vi "GA_Encode.vi"(6 "Parameters":T1={"Population size"=100, "Generations no."=500, "Significant digits"=4, "Crossover probabality"=0.85, "Mutation mode"=enum."one-point, fixed rate", "Use Gray code?"=FALSE, "Mutation rate"=0.05, "Min mutation rate"=0.0005, "Max mutation rate"=0.25, "Reproduction plan"=enum."Steady-state-replace-worst", "Elitism"=FALSE, "Fmax"=1} {"Max mutation rate" min=0.0 max=1.0; "Min mutation rate" min=0.0 max=1.0; "Mutation rate" min=0.0 max=1.0; "Crossover probabality" min=0.0 max=1.0; "Significant digits" min=1; "Generations no." min=1; "Population size" min=1}, 11 "Phenotype":i32[](array[numeric])) -> (3 "Genotype":i8[](array[numeric]))   [LabVIEW 2016, in "Optimal Frequency Bands Search.lvlib" / "GeneticAlgorithm.lvlib"]
doc: "Преобразовать фенотип в генотип. Возможно кодирование генома с помощью двоичного кода, либо кода Грея"
uses:
  GeneticAlgorithm.lvlib
  GA_tParameters.ctl
panel:
  # "This VI is a part of BCI Design library, http://www.ru-bci.org \nCopyright © 2020, Sotnikov Peter, All rights reserved. License: CC BY-NC 4.0"
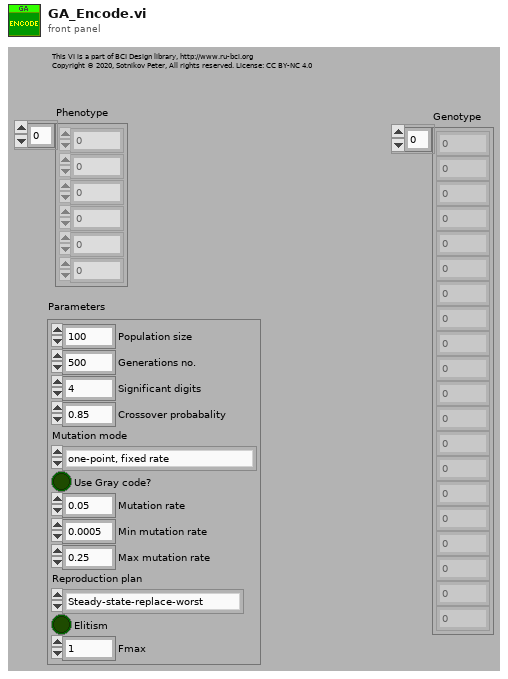
[diagram p1: front panel]
types:
  T1 = typedef "Optimal Frequency Bands Search.lvlib/GeneticAlgorithm.lvlib/GA_tParameters.ctl" = cluster{"Population size":i32, "Generations no.":i32, "Significant digits":i32, "Crossover probabality":dbl, "Mutation mode":enum16{"one-point, fixed rate", "one-point, fitness-adjustable rate", "one-point, distance-adjustable rate"}, "Use Gray code?":bool, "Mutation rate":dbl, "Min mutation rate":dbl, "Max mutation rate":dbl, "Reproduction plan":enum16{"Full generational replacement", "Steady-state-replace-random", "Steady-state-replace-worst"}, "Elitism":bool, "Fmax":i32}
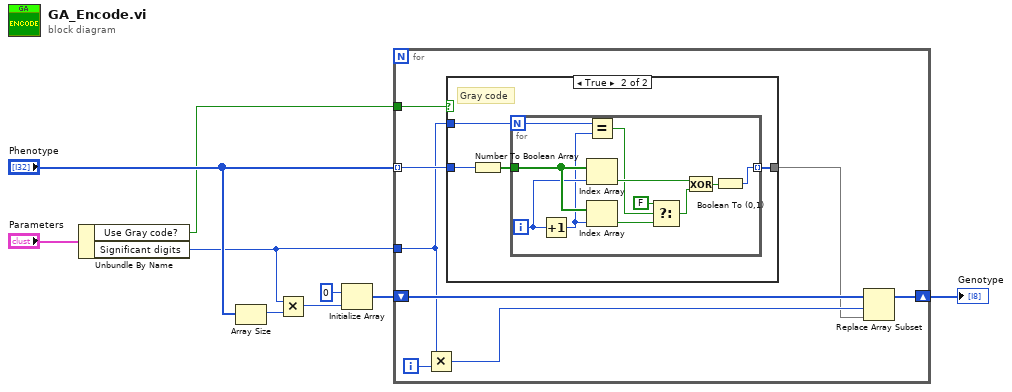
[diagram p0: block diagram]
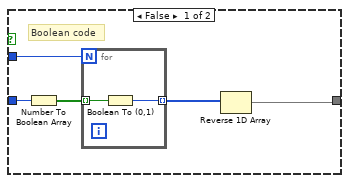
[diagram p2: hidden frame]
diagram:
  n1 = Unbundle By Name("Parameters") -> ("Use Gray code?"=w1:bool, "Significant digits"=w2:i32)
  n2 = Array Size(array="Phenotype") -> (size(s)=w9:i32)
  n3 = Multiply(x=w2, y=w9) -> (x*y=w8:i32)
  n4 = Initialize Array(i8 0 ("element"), w8) -> (w6:i8[])
  n5 = for {
    tunnel: "Phenotype" -> [w13] mode=indexing
    shift-right: [w14] -> w3
    shift-left: w6 -> [w16]
    tunnel: w2 -> [w12]
    tunnel: w1 -> [w10]
    i -> [w17]
    n6 = Multiply(x=w12, y=w17) -> (x*y=w15:i32)
    n7 = case shown="True" w10 {
      tunnel: w13 -> [w22 w28]
      tunnel: w12 -> [w20 w26]
      tunnel: [w18 w25] -> w11
      frame False {
        # "Boolean code"
        n8 = Number To Boolean Array(number=w22) -> (Boolean array=w21:bool[])
        n9 = for {
          N: w20 -> [_]
          tunnel: w21 -> [w24] mode=indexing
          tunnel: [w23] -> w19 mode=indexing
          n10 = Boolean To (0,1)(Boolean=w24) -> (0, 1=w23:i16)
        }
        n11 = Reverse 1D Array(array=w19) -> (reversed array=w18:i16[])
      }
      frame True {
        # "Gray code"
        n12 = Number To Boolean Array(number=w28) -> (Boolean array=w27:bool[])
        n13 = for {
          N: w26 -> [w36]
          tunnel: w27 -> [w39]
          tunnel: [w29] -> w25 mode=indexing
          i -> [w38]
          n14 = Increment(x=w38) -> (x+1=w35:i32)
          n15 = Equal?(x=w36, y=w35) -> (x = y?=w33:bool)
          n16 = Index Array(array=w39, index=w38) -> (element=w37:bool)
          n17 = Index Array(array=w39, index=w35) -> (element=w32:bool)
          n18 = Select(t=FALSE, s=w33, f=w32) -> (s? t:f=w34:bool)
          n19 = Exclusive Or(1:w34, 2:w37) -> (0:w30:bool)
          n20 = Boolean To (0,1)(Boolean=w30) -> (0, 1=w29:i16)
        }
      }
    }
    n21 = Replace Array Subset(array=w16, new element=w11, index=w15) -> (w14:i8[])
  }
  "Genotype" <- w3
